vi "Fingerprint Length.vi"(8 "Error In":errorcluster, 10 "Type":T1=2 items=["MD5"=1, "SHA1"=2], 11 "Session In":refnum<class "Session.lvclass">) -> (0 "Error Out":errorcluster, 2 "Length":i32, 3 "Sesssion Out":refnum<class "Session.lvclass">)   [LabVIEW 2018, in "Toolkit.lvlib" / "Session.lvclass"]
uses:
  Session.lvclass
  API/Typedefs/Host Key Hash Types.ctl
  Session.lvclass/Session.ctl
  SSH/SSH.lvclass/SSH.ctl
  Toolkit.lvlib
  SSH/SSH.lvclass
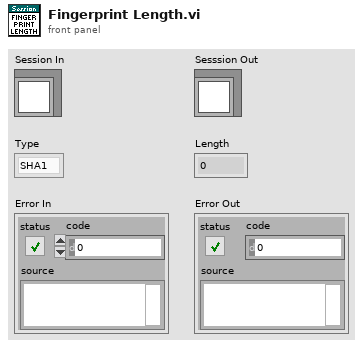
[diagram p1: front panel]
types:
  T1 = typedef "Toolkit.lvlib/Session.lvclass/Host Key Hash Types.ctl" = i32
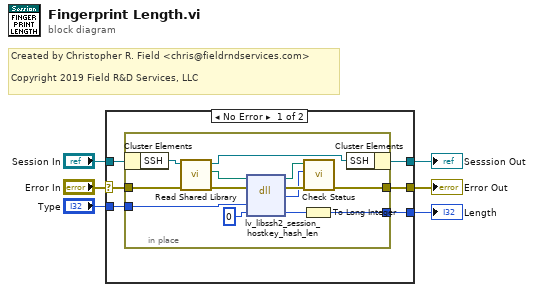
[diagram p0: block diagram]
diagram:
  # "Created by Christopher R. Field <chris@fieldrndservices.com>\n\nCopyright 2019 Field R&D Services, LLC"
  n1 = case shown="No Error" "Error In" {
    selector: "Error In" -> [w12 w27]
    tunnel: [w9 w27] -> w5
    tunnel: "Session In" -> [w11 w26]
    tunnel: [w10 w26] -> w3
    tunnel: [w8 _] -> w2
    tunnel: "Type" -> [w7 _]
    frame No Error {
      n2 = in-place {
        in-place-border: w12 -> [w22]
        in-place-border: [w20] -> w9
        in-place-border: [w18] -> w8
        in-place-border: w7 -> [w13]
        n3 = in-place-cluster #1(w11) -> ("SSH"=w16:refnum<class "SSH.lvclass">)
        n4 = call "Read Shared Library.vi"("Error In"=w22, "SSH In"=w16) -> ("Error Out"=w17:errorcluster, "lv-libssh2 Shared Library"=w14:path, "SSH Out"=w15:refnum<class "SSH.lvclass">)  [unwired: 7 in]
        n5 = dll-call lib="D:/Users/cfield/Code/Field R&D Services/SSH/LabSSH2/LabVIEW/trunk/src/Toolkit/Support/lv-libssh2.*" fn="lv_libssh2_session_hostkey_hash_len"(path in=w14, error in=w17, "type"=w13, "length"=u64 0) -> (path out=w24:path, error out=w25:errorcluster, "result"=w23:i32, "length"=w19:u64)  [unwired: 2 in]
        n6 = To Long Integer(number=w19) -> (32bit integer=w18:i32)
        n7 = call "Check Status.vi"("Error In"=w25, "Status"=w23, "lv-libssh2 Shared Library In"=w24) -> ("Error Out"=w20:errorcluster)  [unwired: 7 in, 1 out]
        n8 = in-place-cluster #1("SSH"=w15) -> (w10:refnum<class "Session.lvclass">)
      }
    }
    frame Error {
    }
  }
  "Sesssion Out" <- w3
  "Error Out" <- w5
  "Length" <- w2
